vi "TreeTesting.vi"() -> ()   [LabVIEW 2019]
uses:
  Tree.lvclass
panel:
  out "Root":variant
  out "Levels 2":u32
  out "x = y?":bool
  out "Root 2":variant
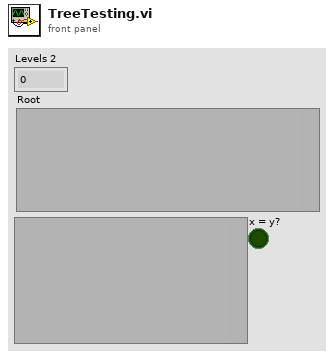
[diagram p1: front panel]
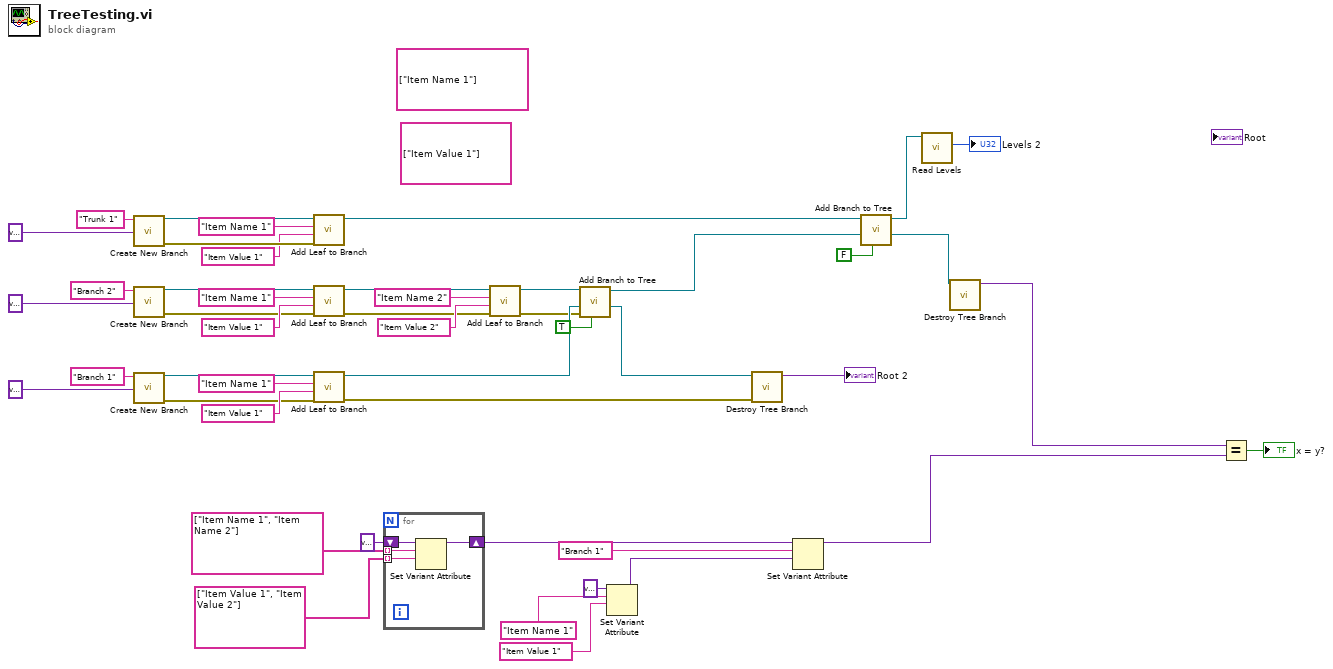
[diagram p0: block diagram]
diagram:
  (unwired) string[] ["Item Value 1"]
  (unwired) string[] ["Item Name 1"]
  n1 = call "Create New Branch.vi"("Branch Data"=variant, "Name"="Trunk 1") -> ("error out"=w15:errorcluster, "Tree out"=w10:refnum<class "Tree.lvclass">)  [unwired: 8 in]
  n2 = call "Create New Branch.vi"("Branch Data"=variant, "Name"="Branch 2") -> ("error out"=w18:errorcluster, "Tree out"=w38:refnum<class "Tree.lvclass">)  [unwired: 8 in]
  n3 = call "Create New Branch.vi"("Branch Data"=variant, "Name"="Branch 1") -> ("error out"=w19:errorcluster, "Tree out"=w47:refnum<class "Tree.lvclass">)  [unwired: 8 in]
  n4 = call "Add Leaf to Branch.vi"("error in"=w15, "Item"="Item Value 1" ("Name"), "Name"="Item Name 1", "Tree in"=w10) -> ("Tree out"=w9:refnum<class "Tree.lvclass">)  [unwired: 6 in, 1 out]
  n5 = call "Add Leaf to Branch.vi"("error in"=w18, "Item"="Item Value 1" ("Name"), "Name"="Item Name 1", "Tree in"=w38) -> ("error out"=w20:errorcluster, "Tree out"=w35:refnum<class "Tree.lvclass">)  [unwired: 6 in]
  n6 = call "Add Leaf to Branch.vi"("error in"=w19, "Item"="Item Value 1" ("Name"), "Name"="Item Name 1", "Tree in"=w47) -> ("error out"=w17:errorcluster, "Tree out"=w33:refnum<class "Tree.lvclass">)  [unwired: 6 in]
  n7 = for {
    tunnel: string[] ["Item Name 1", "Item Name 2"] -> [w51] mode=indexing
    tunnel: string[] ["Item Value 1", "Item Value 2"] -> [w50] mode=indexing
    shift-right: [w48] -> w27
    shift-left: variant -> [w49]
    n8 = Set Variant Attribute(Variant=w49, name=w51, value=w50) -> (Variant out=w48:variant)  [unwired: 1 in, 2 out]
  }
  n9 = call "Add Leaf to Branch.vi"("error in"=w20, "Item"="Item Value 2" ("Name"), "Name"="Item Name 2", "Tree in"=w35) -> ("error out"=w21:errorcluster, "Tree out"=w34:refnum<class "Tree.lvclass">)  [unwired: 6 in]
  n10 = call "Add Branch to Tree.vi"("Truncate Branch?"=TRUE, "error in"=w21, "Branch in"=w33, "Root in"=w34) -> ("Branch out"=w32:refnum<class "Tree.lvclass">, "Root out"=w6:refnum<class "Tree.lvclass">)  [unwired: 5 in, 1 out]
  n11 = Set Variant Attribute(Variant=variant ("variant"), name="Item Name 1", value="Item Value 1") -> (Variant out=w26:variant)  [unwired: 1 in, 2 out]
  n12 = call "Destroy Tree Branch.vi"("error in"=w17, "Tree in"=w32) -> ("Root"=→"Root 2":variant)  [unwired: 8 in, 1 out]
  n13 = Set Variant Attribute(Variant=w27, name="Branch 1", value=w26) -> (Variant out=w16:variant)  [unwired: 1 in, 2 out]
  n14 = call "Add Branch to Tree.vi"("Truncate Branch?"=FALSE, "Branch in"=w6, "Root in"=w9) -> ("Branch out"=w3:refnum<class "Tree.lvclass">, "Root out"=w8:refnum<class "Tree.lvclass">)  [unwired: 6 in, 1 out]
  n15 = call "Read Levels.vi"("Tree in"=w8) -> ("Levels"=→"Levels 2":u32)  [unwired: 8 in, 2 out]
  n16 = call "Destroy Tree Branch.vi"("Tree in"=w3) -> ("Root"=w1:variant)  [unwired: 9 in, 1 out]
  n17 = Equal?(x=w1, y=w16) -> (x = y?=→"x = y?":bool)
